vi "cRIOControllerInfo.vi"(8 "error in (no error)":errorcluster, 11 "session in":refnum<k21>="localhost") -> (0 "error out":errorcluster, 2 "cRIO Controller Information":T1)   [LabVIEW 2017, in "cRIODetectHW.lvlib"]
doc: "Gets information about the cRIO controller, such as model name, model code, serial number, MAC address, host name, and IP address."
uses:
  <vilib>/addons/cRIODetectHW/cRIODetectHW.lvlib
  <vilib>/addons/cRIODetectHW/control/cRIO Product Info.ctl
  <vilib>/nisyscfg/Initialize (Control).vi
  <vilib>/nisyscfg/Find Hardware.vi
  <vilib>/nisyscfg/Close (Hardware).vi
  <vilib>/nisyscfg/Close (Filter).vi
  <vilib>/nisyscfg/Close (System).vi
  <vilib>/nisyscfg/nisyscfg.lvlib
  <resource>/objmgr/nicontrollersysapi.rc
  <resource>/objmgr/niflexrioatomicsae.rc
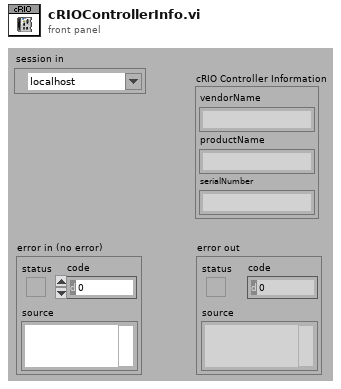
[diagram p1: front panel]
types:
  T1 = typedef "cRIODetectHW.lvlib/cRIO Product Info.ctl" = cluster{"vendorName":string, "productName":string, "serialNumber":string}
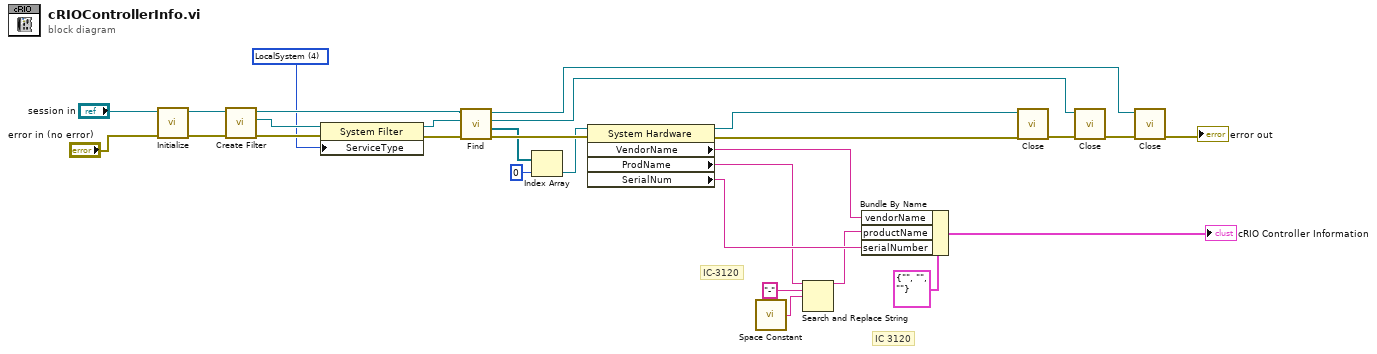
[diagram p0: block diagram]
diagram:
  w16 = u32 4 items=["mDnsNiTcp", "mDnsNiRealtime", "mDnsNiSysapi", "mDnsNiHttp", "LocalSystem", "LocalNetInterface", "LocalTimeKeeper", "LocalTimeSource", "mDnsLxi"] ("Service Type")
  # "IC 3120"
  # "IC-3120"
  n1 = call-poly <vilib>:"Initialize.vi"("error in (no error)"="error in (no error)", "Target (localhost)"="session in") -> ("error out"=w24:errorcluster, "Session out"=w15:refnum<k21>)  [unwired: 7 in, 1 out]
  n2 = call <vilib>:"Create Filter.vi"("error in (no error)"=w24, "Session in"=w15) -> ("error out"=w25:errorcluster, "Filter out"=w26:refnum<k20>, "Session out"=w23:refnum<k21>)  [unwired: 7 in]
  n3 = property class="System Filter"(reference=w26, error in=w25, "ServiceType"=w16) -> (reference out=w20:refnum<k20>, error out=w21:errorcluster)
  n4 = call-poly <vilib>:"Find.vi"("error in (no error)"=w21, "Filter in"=w20, "Session in"=w23) -> ("error out"=w19:errorcluster, "Resources out"=w9:refnum<k20>[], "Filter out"=w17:refnum<k20>, "Session out"=w22:refnum<k21>)  [unwired: 5 in]
  n5 = Index Array(array=w9, index=0) -> (element=w8:refnum<k20>)
  n6 = property class="System Hardware"(reference=w8, error in=w19) -> (reference out=w10:refnum<k20>, error out=w11:errorcluster, "VendorName"=w6:string, "ProdName"=w4:string, "SerialNum"=w5:string)
  n7 = call <vilib>:"Space Constant.vi"() -> ("String"=w1:string)
  n8 = Search and Replace String(input string=w4, search string="-", replace string=w1) -> (result string=w3:string)  [unwired: 5 in, 3 out]
  n9 = Bundle By Name(cluster=T1 {"vendorName"="", "productName"="", "serialNumber"=""} ("cRIO Controller Info"), "vendorName"=w6, "productName"=w3, "serialNumber"=w5) -> (→"cRIO Controller Information":T1)
  n10 = call-poly <vilib>:"Close.vi"("error in (no error)"=w11, "Resource in"=w10) -> ("error out"=w18:errorcluster)  [unwired: 9 in]
  n11 = call-poly <vilib>:"Close.vi"("error in (no error)"=w18, "Filter in"=w17) -> ("error out"=w12:errorcluster)  [unwired: 9 in]
  n12 = call-poly <vilib>:"Close.vi"("error in (no error)"=w12, "Session in"=w22) -> ("error out"=→"error out":errorcluster)  [unwired: 9 in]
